vi "Ping Test.vi"(8 "error in (no error)":errorcluster, 11 "IP Address to Ping":string) -> (0 "error out":errorcluster, 2 "Command Prompt Output":string, 3 "Ping Success?":bool)   [LabVIEW 2025]
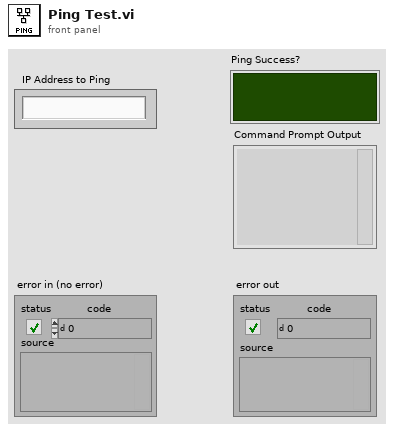
[diagram p1: front panel]
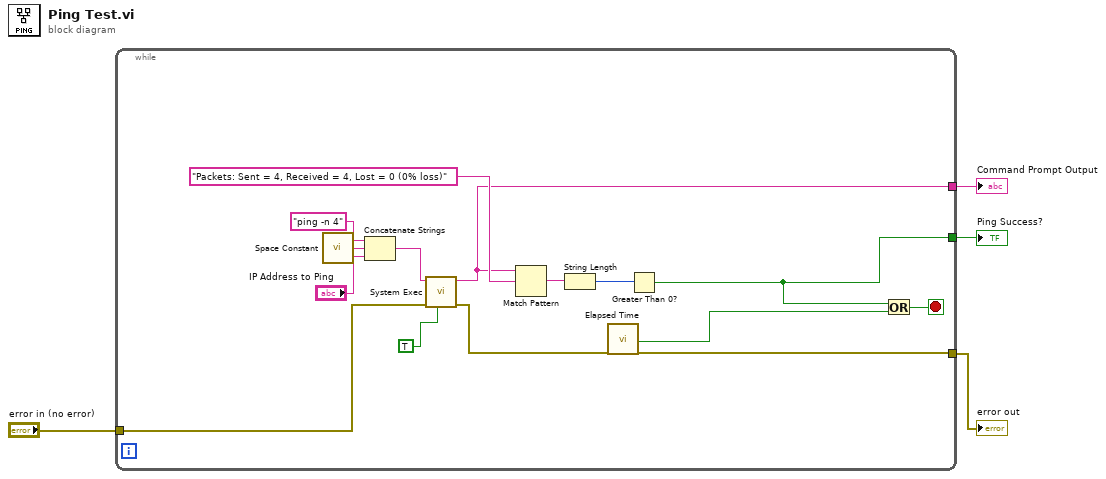
[diagram p0: block diagram]
diagram:
  n1 = while {
    tunnel: [w7] -> w2
    tunnel: [w10] -> w4
    tunnel: "error in (no error)" -> [w6]
    tunnel: [w5] -> w1
    stop <- w19 stop-if-true
    n2 = call <vilib>:"Space Constant.vi"() -> ("String"=w15:string)
    n3 = Concatenate Strings("ping -n 4", w15, "IP Address to Ping") -> (w17:string)
    n4 = call <vilib>:"System Exec.vi"("run minimized? (F)"=TRUE, "error in (no error)"=w6, "command line"=w17) -> ("error out"=w8:errorcluster, "standard output"=w5:string)  [unwired: 5 in, 2 out]
    n5 = Match Pattern(string=w5, regular expression="Packets: Sent = 4, Received = 4, Lost = 0 (0% loss)") -> (match substring=w13:string)  [unwired: 1 in, 3 out]
    n6 = String Length(string=w13) -> (length=w11:i32)
    n7 = call "Elapsed Time"("error in (no error)"=w8) -> ("Time has Elapsed"=w9:bool, "error out"=w7:errorcluster)  [unwired: 11 in, 6 out]
    n8 = Greater Than 0?(x=w11) -> (x > 0?=w10:bool)
    n9 = Or(x=w10, y=w9) -> (x .or. y?=w19:bool)
  }
  "Ping Success?" <- w4
  "error out" <- w2
  "Command Prompt Output" <- w1
